vi "Set Temp Thold Arrays.vi"(11 "Set Temperature Threshold Arrays":T1) -> ()   [LabVIEW 2015, in "Tool Module.lvlib"]
uses:
  Tool Module.lvlib
  Tool Typedefs/_Temperature Threshold Arrays--typedef.ctl
  ToolModGLOB.vi
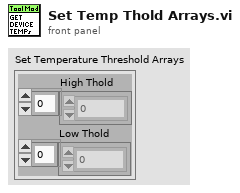
[diagram p1: front panel]
types:
  T1 = typedef "_Temperature Threshold Arrays--typedef.ctl" = cluster{"High Thold ":dbl[], "Low Thold ":dbl[]}
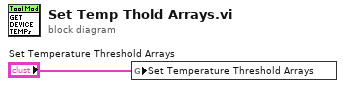
[diagram p0: block diagram]
diagram:
  n1 = global write "ToolModGLOB.vi" "Set Temperature Threshold Arrays"("Set Temperature Threshold Arrays") -> ()
